vi "GDSArray_RemoveDublicatesInArray.vi"(0 "Strings in":string[](array[string]), 1 "Paths in":path[](array[path]), 5 "error in (no error)":errorcluster) -> (14 "Strings out":string[](array[string]), 15 "Paths out":path[](array[path]), 19 "error out":errorcluster)   [LabVIEW 2020]
doc: "-"
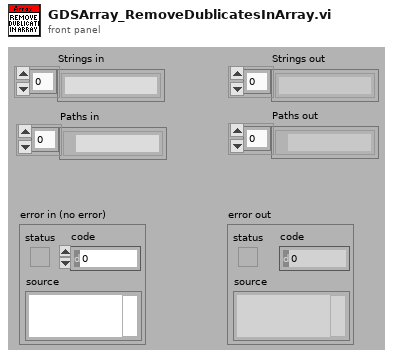
[diagram p1: front panel]
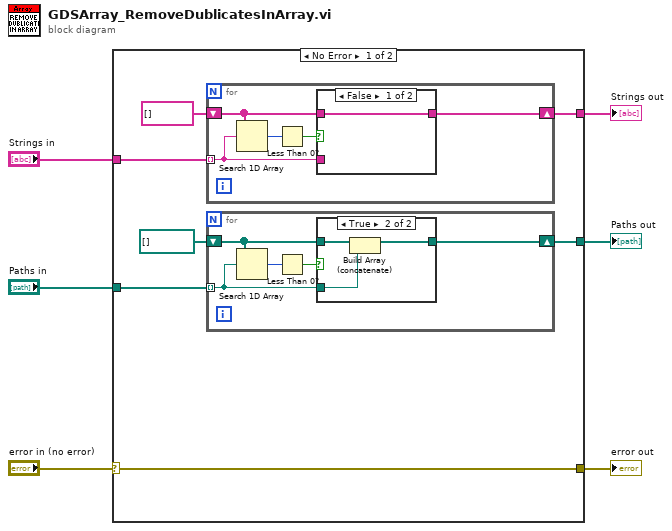
[diagram p0: block diagram]
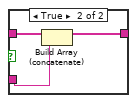
[diagram p3: hidden frame]
diagram:
  n1 = case shown="No Error" "error in (no error)" {
    selector: "error in (no error)" -> [w13 w34]
    tunnel: [w13 w34] -> w5
    tunnel: "Strings in" -> [w11 w33]
    tunnel: [w10 w33] -> w3
    tunnel: "Paths in" -> [w8 w32]
    tunnel: [w7 w32] -> w1
    frame No Error {
      n2 = for {
        shift-right: [w23] -> w10
        shift-left: string[] [] ("Arrayout") -> [w25]
        tunnel: w11 -> [w24] mode=indexing
        n3 = Search 1D Array(1D array=w25, element=w24) -> (index of element=w27:i32)  [unwired: 1 in]
        n4 = Less Than 0?(x=w27) -> (x < 0?=w26:bool)
        n5 = case shown="False" w26 {
          tunnel: w25 -> [w28 w31]
          tunnel: w24 -> [_ w30]
          tunnel: [w28 w29] -> w23
          frame False {
          }
          frame True {
            n6 = Build Array (concatenate)(w31, w30) -> (w29:string[])
          }
        }
      }
      n7 = for {
        shift-right: [w14] -> w7
        shift-left: path[] [] ("Arrayout") -> [w16]
        tunnel: w8 -> [w15] mode=indexing
        n8 = Search 1D Array(1D array=w16, element=w15) -> (index of element=w18:i32)  [unwired: 1 in]
        n9 = Less Than 0?(x=w18) -> (x < 0?=w17:bool)
        n10 = case shown="True" w17 {
          tunnel: w16 -> [w19 w22]
          tunnel: w15 -> [_ w21]
          tunnel: [w19 w20] -> w14
          frame False {
          }
          frame True {
            n11 = Build Array (concatenate)(w22, w21) -> (w20:path[])
          }
        }
      }
    }
    frame Error {
    }
  }
  "error out" <- w5
  "Strings out" <- w3
  "Paths out" <- w1
